vi "FRIC_navX_Internal_I2C_ProcessingLoop.vi"(7 "Device Number":T2, 10 "I2C Bus":T1=enum."I2C MXP", 11 "Rate (4Hz-200Hz)":u8=50 min=4 max=200) -> ()   [LabVIEW 2018]
doc: "This navX VI handles the reading/writing for the navX. All of the good stuff is in here.\nTHIS VI SHOULD NOT BE CALLED BY THE USER!"
uses:
  <vilib>/Rock Robotics/SystemInterfaces/i2clib/i2c_bus.ctl
  _TypeDefs/FRIC_navX_DeviceNumbersTypeDef.ctl
  _TypeDefs/FRIC_navX_ProcessingLoopStatesTypeDef_I2C.ctl
  _TypeDefs/FRIC_navX_I2C Process Loop TypeDef.ctl
  _TypeDefs/Z900_navX_DeviceTypeDef.ctl
  _TypeDefs/Z900_navX_ProtocolTypeDef.ctl
  _TypeDefs/Z900_navX_NotifyPacketTypeDef.ctl
  _TypeDefs/Z900_navX_ActionTypeDef.ctl
  _TypeDefs/Z900_navX_SerialStreamTypeDef.ctl
  _TypeDefs/Z900_navX_IntegrationControlRegisters.ctl
  <vilib>/Rock Robotics/WPI/SPI/WPI_SPIDevRef.ctl
  <vilib>/Rock Robotics/SystemInterfaces/spilib/spi_bus.ctl
  <vilib>/Rock Robotics/WPI/SerialPort/WPI_SerialPort.ctl
  <vilib>/Rock Robotics/WPI/SerialPort/WPI_SerialPortRef.ctl
  <vilib>/Platform/TimedLoop/XDataNode/timing_clust.ctl
  <vilib>/Platform/TimedLoop/XDataNode/nitl_modes.ctl
  <vilib>/Platform/TimedLoop/XDataNode/wakeup.ctl
  _TypeDefs/Z900_navX_DeviceRegisters.ctl
  _TypeDefs/Flags/Z900_navX_Flags_CapabilityTypeDef.ctl
  _Util/Z900_navX_Util_LittleEndian_to_BigEndian.vi
  <vilib>/Rock Robotics/SystemInterfaces/Utilities/FPGA_UtilitiesRead LocalTime.vi
  <vilib>/Platform/TimedLoop/XDataNode/XDataNode.xnode
  <vilib>/Platform/TimedLoop/XDataNode/XDNodeRunTimeDep.lvlib
panel:
  in  "Tab Control":enum32{"Page 1", "Page 2"}(tab)
  in  "Halt":bool
  out "Connected":bool
  out "error":errorcluster
  out "Loop Time":i64
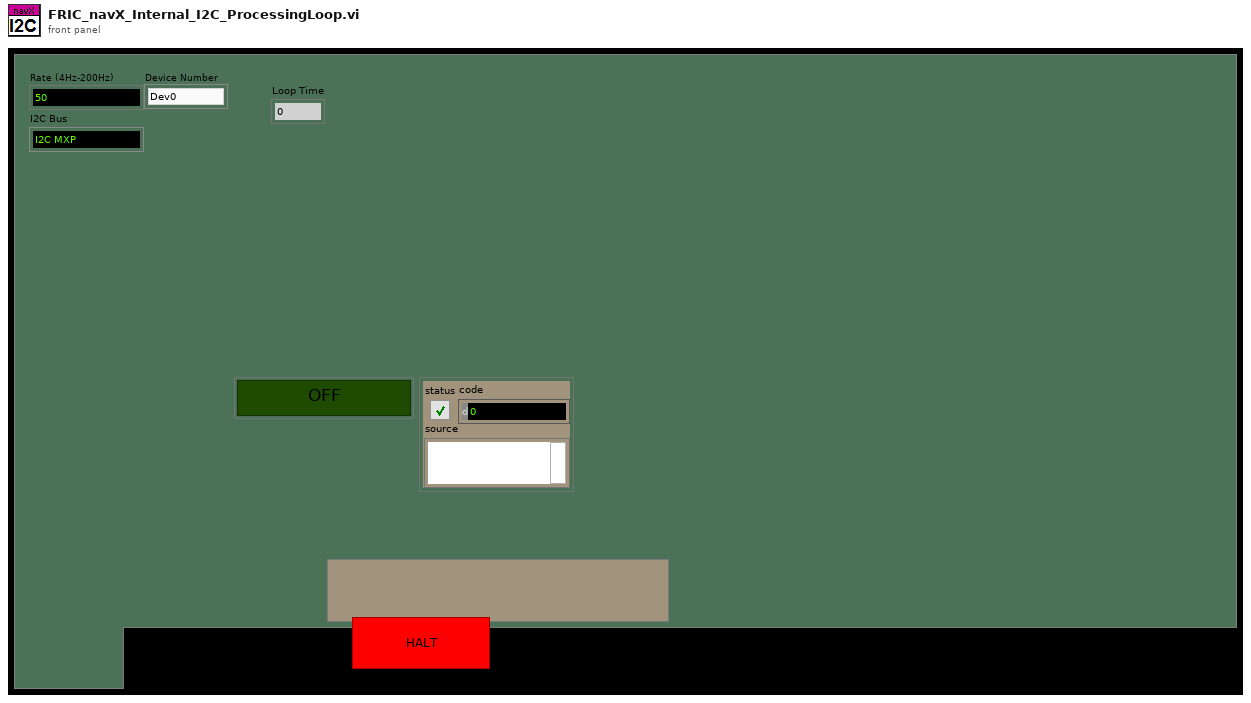
[diagram p1: front panel]
types:
  T1 = typedef "i2c_bus.ctl" = enum16{"I2C On-Board", "I2C MXP", "Invalid"}
  T2 = typedef "FRIC_navX_DeviceNumbersTypeDef.ctl" = enum16{"Dev0", "Dev1", "Dev2", "Dev3"}
  T3 = typedef "FRIC_navX_I2C Process Loop TypeDef.ctl" = cluster{"State Array":T4[], "error":errorcluster, "FPGA Cluster":cluster{"Last Valid FPGA Time":dbl, "Error Count":i32, "Initialized":bool}, "Device Info":T5, "I2CDevRef":cluster{"DevStatus":errorcluster, "Device Address":u8, "Handle":i32, "I2C Bus":T1}, "Registry":u8[], "Command Array":T7[], "Connected?":bool, "navX Device Memory Size":i32, "notification":T8, "Memory Size Set":bool, "SPIDevRef":T11, "navX Serial Open":cluster{"Stream Type":T10, "Serial Port":T13}, "SerialPortRef":T14, "Serial Read Buffer":string, "Serial Write Buffer":string[], "Device Number":T2, "navX SPI Open":cluster{"SPI Bus":T12, "Clock Rate (Hz)":dbl}, "Loop dt":i64, "current time":timestamp, "Loop Time":i64}
  T4 = typedef "FRIC_navX_ProcessingLoopStatesTypeDef_I2C.ctl" = enum16{"Process", "INI", "Check Packets Valid", "Close", "Clear VISA", "Generate Command", "Last Packet Valid", "Open", "Read", "Reset Serial", "Set Termination Char", "Update AE", "Wait", "Write", "Exit"}
  T5 = typedef "Z900_navX_DeviceTypeDef.ctl" = cluster{"Interface":cluster{"Protocol":T6, "Update Rate (4Hz-200Hz)":u8, "navX Open TypeDef":variant}, "Notify Packet":refnum<notifier>, "Loop VI Refnum":refnum<vi>, "Ready to Close Occurrence Refnum":refnum<k4>, "Name":string}
  T6 = typedef "Z900_navX_ProtocolTypeDef.ctl" = enum16{"SERIAL", "I2C", "SPI"}
  T7 = typedef "Z900_navX_IntegrationControlRegisters.ctl" = u8
  T8 = typedef "Z900_navX_NotifyPacketTypeDef.ctl" = cluster{"navX Action":T9, "Data":variant, "Stream Type":T10, "Device Number":T2}
  T9 = typedef "Z900_navX_ActionTypeDef.ctl" = enum16{"None", "Halt", "Normal Read", "Update Serial Protocol", "Update Rate Htz", "Zero-Yaw", "Zero-Displacement", "Zero-Velocity"}
  T10 = typedef "Z900_navX_SerialStreamTypeDef.ctl" = enum16{"YRPH", "Quaterinons", "Gyro/Raw", "AHRS", "AHRSAndPositioning", "AHRSAndPOSTime"}
  T11 = typedef "WPI_SPIDevRef.ctl" = cluster{"DevStatus":errorcluster, "Handle":i32, "SPI Bus":T12}
  T12 = typedef "spi_bus.ctl" = enum16{"SPI On-Board, CS0", "SPI On-Board, CS1", "SPI On-Board, CS2", "SPI On-Board, CS3", "SPI MXP", "Invalid"}
  T13 = typedef "WPI_SerialPort.ctl" = enum16{"Onboard RS-232", "MXP TTL", "USB 1", "USB 2"}
  T14 = typedef "WPI_SerialPortRef.ctl" = cluster{"DevStatus":errorcluster, "Serial Port Name":refnum<visa-resource-name>}
  T15 = typedef "XDNodeRunTimeDep.lvlib/timing_clust.ctl" = cluster{"Expected End [f-1]":u64, "Actual End [f-1]":u64, "Finished Late? [f-1]":bool, "Expected End [i-1]":u64, "Actual End [i-1]":u64, "Finished Late? [i-1]":bool, "Expected Start [i]":u64, "Actual Start [i]":u64, "Expected Start [f]":u64, "Actual Start [f]":u64, "Source Name":string, "Structure Name":string, "Period":i64, "Deadline":i64, "Offset":i64, "Start":i64, "Priority":i32, "Timeout":i32, "Mode":T16, "Wakeup Reason":T17, "Error":errorcluster, "Source Type":string, "Secondary Source Type":string, "Global End Time":u64, "Global Start Time":u64, "Frame Duration":u64, "Iteration Duration":u64, "Assigned CPU":i32, "I/O Scan Engine Mode":u32}
  T16 = typedef "XDNodeRunTimeDep.lvlib/nitl_modes.ctl" = enum32{"No Change", "Process missed periods, maintain original phase", "Discard missed periods, maintain original phase", "Process missed periods, ignore original phase", "Discard missed periods, ignore original phase"}
  T17 = typedef "XDNodeRunTimeDep.lvlib/wakeup.ctl" = enum32{"Normal", "Aborted", "Asynchronous wakeup", "Timing source error", "Timed loop error", "Timeout"}
  T18 = typedef "Z900_navX_DeviceRegisters.ctl" = u8
  T19 = typedef "Z900_navX_Flags_CapabilityTypeDef.ctl" = u16
  T20 = cluster{"DevStatus":errorcluster, "Device Address":u8, "Handle":i32, "I2C Bus":T1}
  T21 = cluster{"Last Valid FPGA Time":dbl, "Error Count":i32, "Initialized":bool}
  T22 = typedef "WPI_I2CDevRef.ctl" = cluster{"DevStatus":errorcluster, "Device Address":u8, "Handle":i32, "I2C Bus":T1}
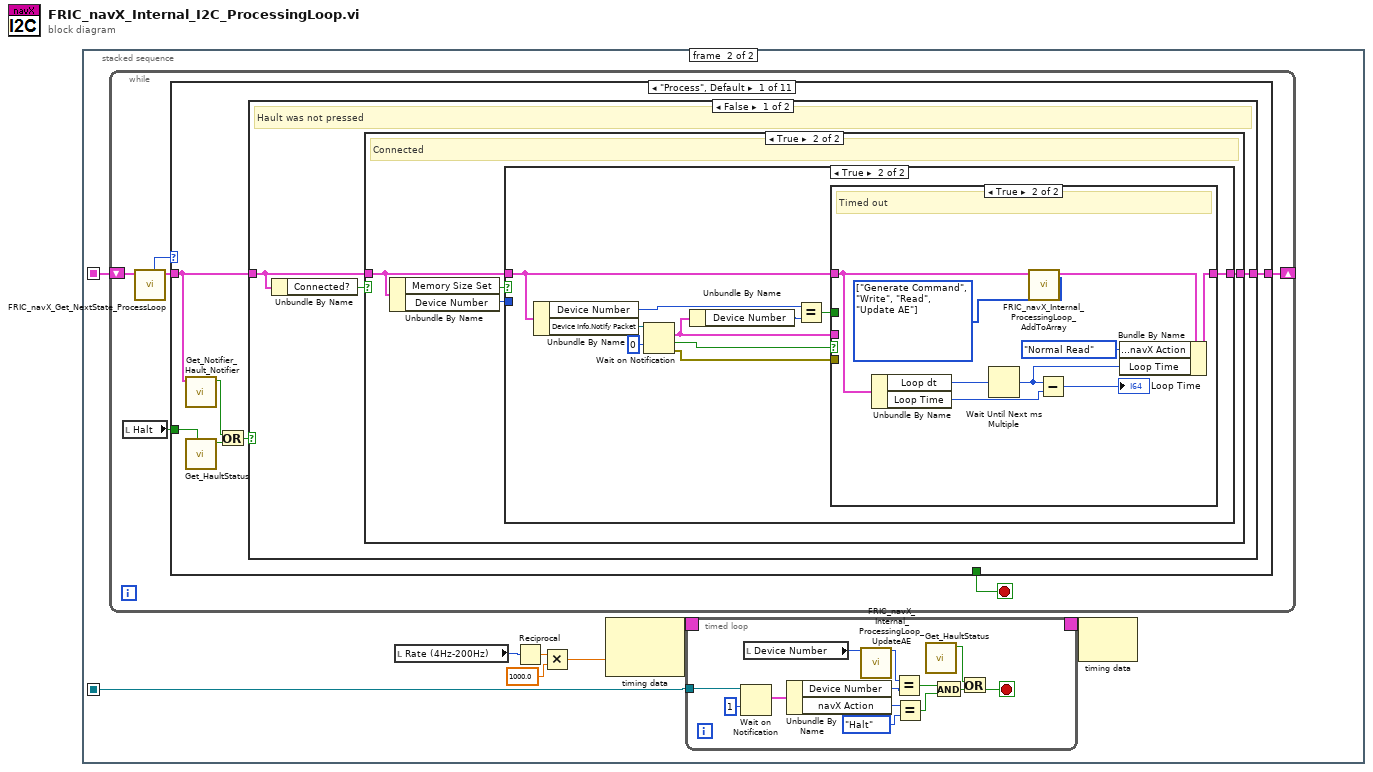
[diagram p0: block diagram]
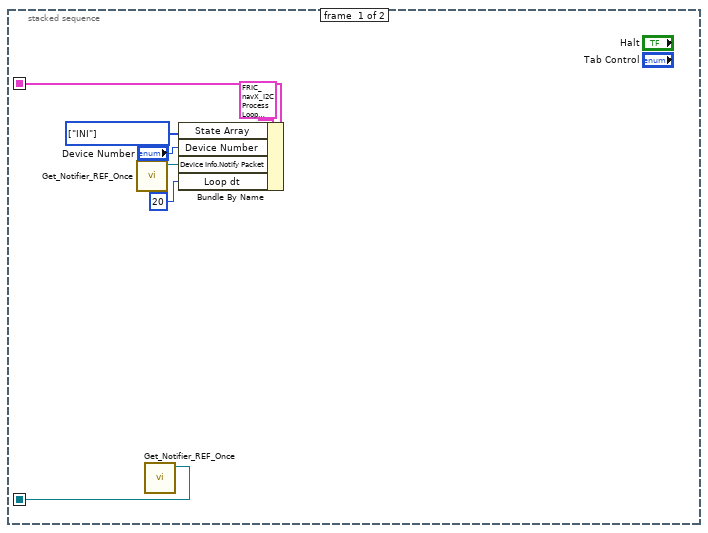
[diagram p2: hidden frame]
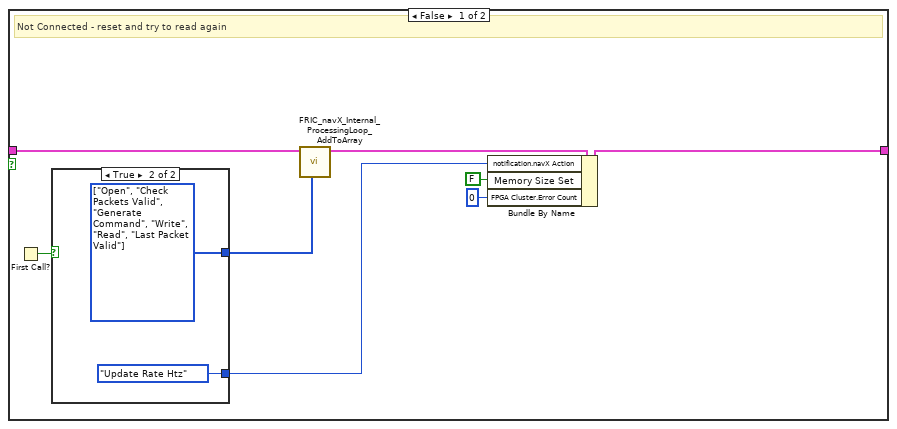
[diagram p3: hidden frame]
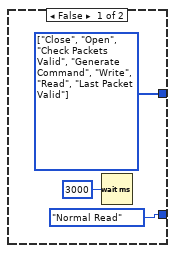
[diagram p4: hidden frame]
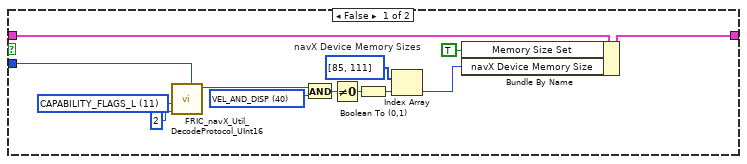
[diagram p5: hidden frame]
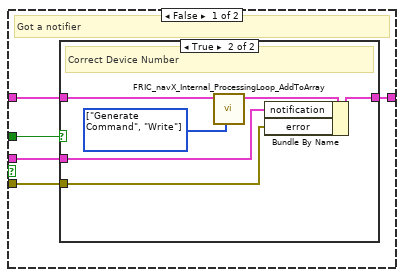
[diagram p6: hidden frame]
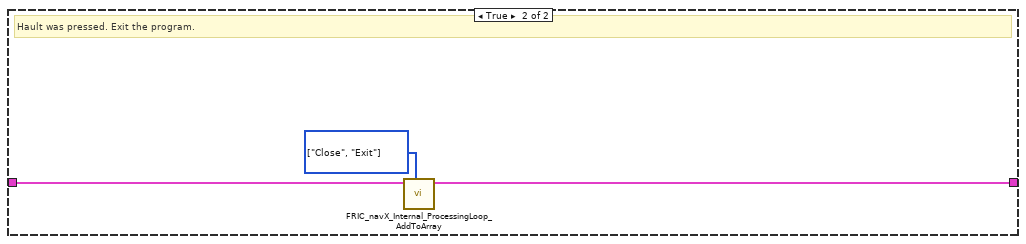
[diagram p8: hidden frame]
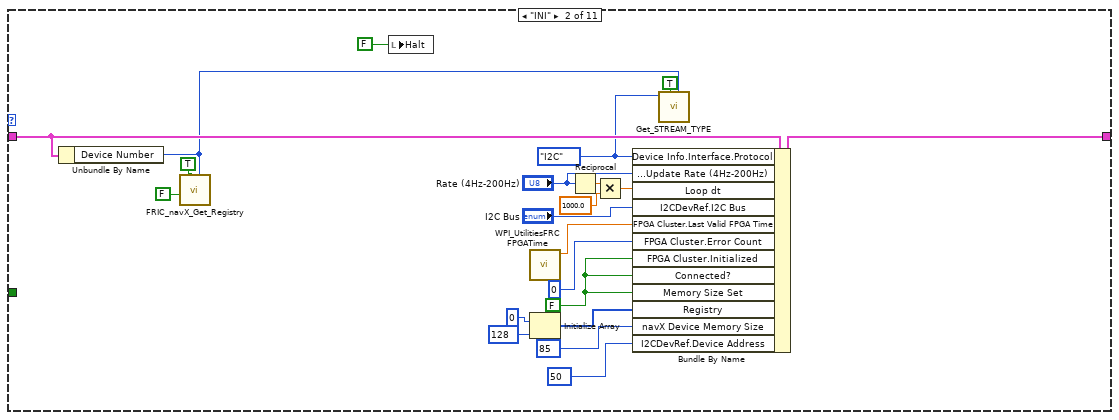
[diagram p9: hidden frame]
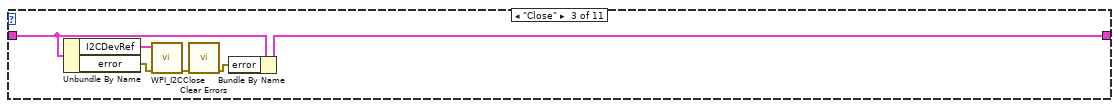
[diagram p10: hidden frame]
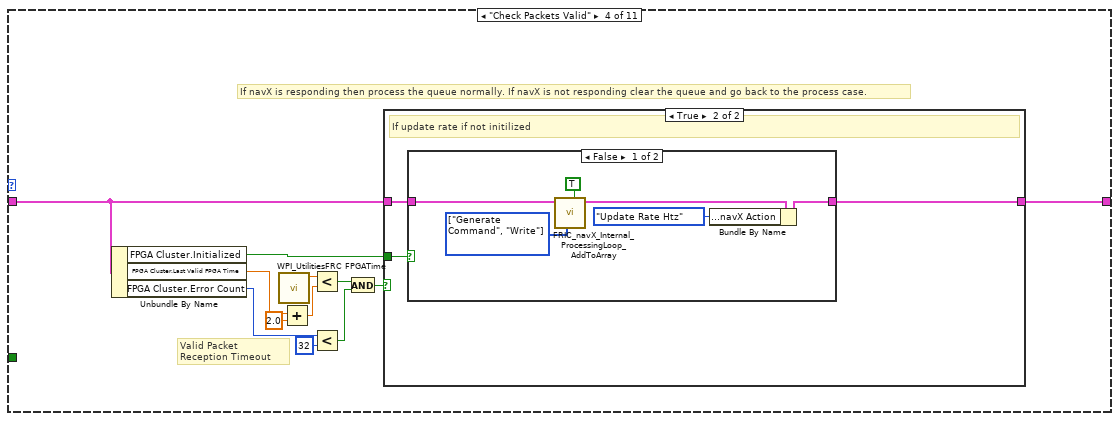
[diagram p11: hidden frame]
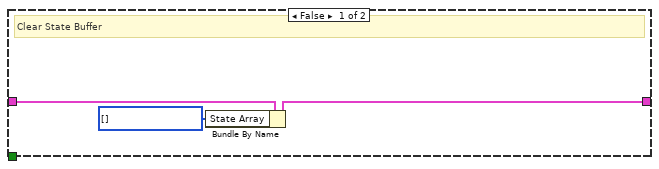
[diagram p12: hidden frame]
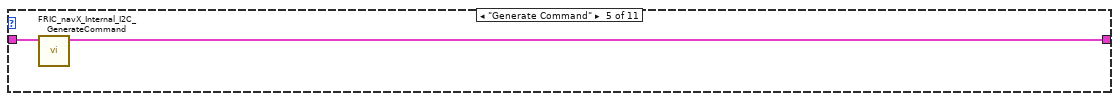
[diagram p14: hidden frame]
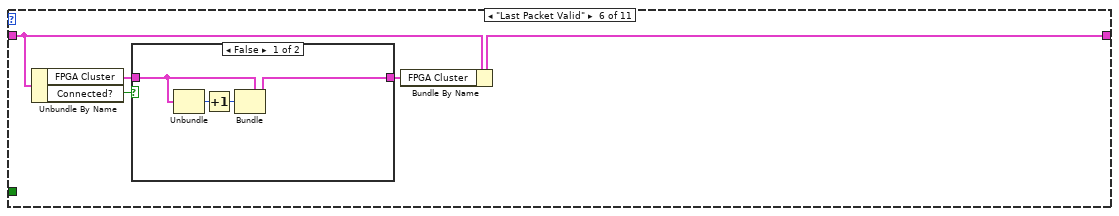
[diagram p15: hidden frame]
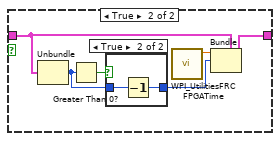
[diagram p16: hidden frame]
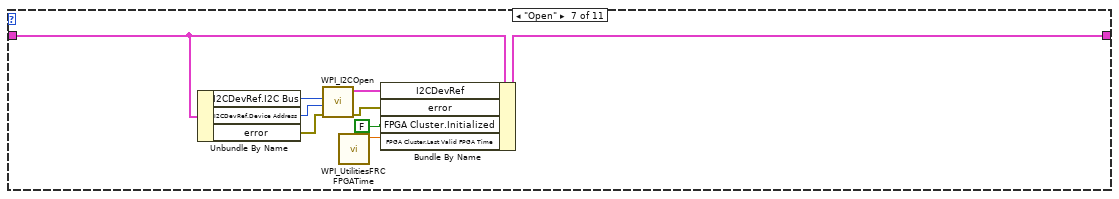
[diagram p18: hidden frame]
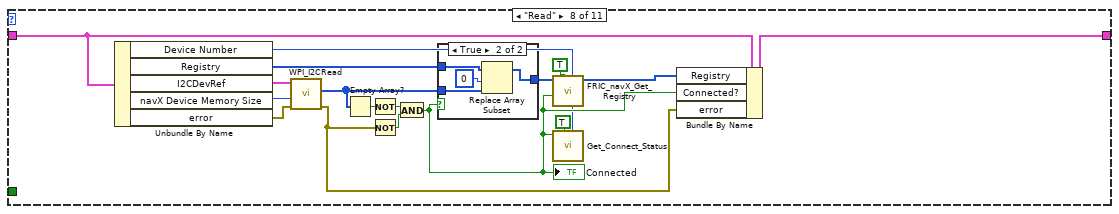
[diagram p19: hidden frame]
diagram:
  n1 = stacked-sequence {
    seq-local: [w7 _] -> [_ w15]
    seq-local: [w1 _] -> [_ w8]
    frame #0 {
      w5 = T4[] [enum."INI"] items=["Process", "INI", "Check Packets Valid", "Close", "Clear VISA", "Generate Command", "Last Packet Valid", "Open", "Read", "Reset Serial", "Set Termination Char", "Update AE", "Wait", "Write", "Exit"] ("State Array")
      n2 = call "Get_Notifier_REF_Once.vi"() -> ("notifier ref out"=w3:refnum<notifier>)  [unwired: 10 in, 1 out]
      n3 = call "Get_Notifier_REF_Once.vi"() -> ("notifier ref out"=w1:refnum<notifier>)  [unwired: 10 in, 1 out]
      n4 = Bundle By Name(cluster=T3 {"State Array"=[enum."INI", enum."Open"], "error"={"status"=FALSE, "code"=0, "source"=""}, "FPGA Cluster"={"Last Valid FPGA Time"=0.0, "Error Count"=0, "Initialized"=FALSE}, "Device Info"={"Interface"={"Protocol"=enum."SERIAL", "Update Rate (4Hz-200Hz)"=4, "navX Open TypeDef"=variant}, "Notify Packet"=refnum, "Loop VI Refnum"=refnum, "Ready to Close Occurrence Refnum"=refnum, "Name"=""}, "I2CDevRef"={"DevStatus"={"status"=FALSE, "code"=0, "source"=""}, "Device Address"=0, "Handle"=0, "I2C Bus"=enum."Invalid"}, "Registry"=[], "Command Array"=[214, 32], "Connected?"=FALSE, "navX Device Memory Size"=85, "notification"={"navX Action"=enum."None", "Data"=variant, "Stream Type"=enum."YRPH", "Device Number"=enum."Dev0"}, "Memory Size Set"=FALSE, "SPIDevRef"={"DevStatus"={"status"=FALSE, "code"=0, "source"=""}, "Handle"=0, "SPI Bus"=enum."SPI On-Board, CS0"}, "navX Serial Open"={"Stream Type"=enum."YRPH", "Serial Port"=enum."Onboard RS-232"}, "SerialPortRef"={"DevStatus"={"status"=FALSE, "code"=0, "source"=""}, "Serial Port Name"=""}, "Serial Read Buffer"="", "Serial Write Buffer"=[], "Device Number"=enum."Dev0", "navX SPI Open"={"SPI Bus"=enum."SPI MXP", "Clock Rate (Hz)"=500000.0}, "Loop dt"=0, "current time"=timestamp(0 s since 1904-01-01), "Loop Time"=0} ("I2C Process Loop TypeDef"), "State Array"=w5, "Device Number"="Device Number", "Device Info.Notify Packet"=w3, "Loop dt"=i64 20) -> (w7:T3)
    }
    frame #1 {
      n5 = while {
        shift-right: [w35] -> _
        shift-left: w15 -> [w38]
        stop <- w39 stop-if-true
        n6 = local read "Halt"() -> (w34:bool)
        n7 = call "FRIC_navX_Get_NextState_ProcessLoop.vi"("I2C Process Loop TypeDef (in)"=w38) -> ("I2C Process Loop TypeDef (out)"=w37:T3, "Current State"=w36:T4)  [unwired: 9 in]
        n8 = case shown="\"Process\", Default" w36 {
          tunnel: [_ _ _ _ _ _ _ _ _ w223 _] -> w39
          tunnel: w37 -> [w44 w123 w137 w144 w166 w170 w192 w205 w221 w225 w233]
          tunnel: [w45 w129 w136 w145 w165 w169 w191 w204 w222 w225 w233] -> w35
          tunnel: w34 -> [w42 _ _ _ _ _ _ _ _ _ _]
          frame "Process", Default {
            n9 = call "Get_Notifier_Hault_Notifier.vi"("Process Loop TypeDef (in)"=w44) -> ("Hault Notifier"=w41:bool)  [unwired: 10 in]
            n10 = call "Get_HaultStatus.vi"("Update"=w42) -> ("Hault"=w40:bool)  [unwired: 10 in]
            n11 = Or(x=w41, y=w40) -> (x .or. y?=w43:bool)
            n12 = case shown="False" w43 {
              tunnel: [w48 w111] -> w45
              tunnel: w44 -> [w46 w112]
              frame False {
                # "Hault was not pressed"
                n13 = Unbundle By Name(w46) -> ("Connected?"=w47:bool)
                n14 = case shown="True" w47 {
                  tunnel: w46 -> [w56 w64]
                  tunnel: [w53 w65] -> w48
                  frame False {
                    # "Not Connected - reset and try to read again"
                    n15 = First Call?() -> (First Call?: T/F=w50:bool)
                    n16 = case shown="True" w50 {
                      tunnel: [w59 w61] -> w55
                      tunnel: [Z900_navX_ActionTypeDef."Normal Read" ("notification.navX Action") Z900_navX_ActionTypeDef."Update Rate Htz" ("notification.navX Action")] -> w49
                      frame False {
                        w59 = T4[] [enum."Close", enum."Open", enum."Check Packets Valid", enum."Generate Command", enum."Write", enum."Read", enum."Last Packet Valid"] items=["Process", "INI", "Check Packets Valid", "Close", "Clear VISA", "Generate Command", "Last Packet Valid", "Open", "Read", "Reset Serial", "Set Termination Char", "Update AE", "Wait", "Write", "Exit"]
                        n17 = Wait (ms)(milliseconds to wait=u32 3000) -> ()  [unwired: 1 out]
                      }
                      frame True {
                        w61 = T4[] [enum."Open", enum."Check Packets Valid", enum."Generate Command", enum."Write", enum."Read", enum."Last Packet Valid"] items=["Process", "INI", "Check Packets Valid", "Close", "Clear VISA", "Generate Command", "Last Packet Valid", "Open", "Read", "Reset Serial", "Set Termination Char", "Update AE", "Wait", "Write", "Exit"]
                      }
                    }
                    n18 = call "FRIC_navX_Internal_ProcessingLoop_AddToArray.vi"("States Array"=w55, "I2C Process Loop TypeDef (in)"=w56) -> ("I2C Process Loop TypeDef (out)"=w54:T3)  [unwired: 9 in]
                    n19 = Bundle By Name(cluster=w54, "notification.navX Action"=w49, "Memory Size Set"=FALSE, "FPGA Cluster.Error Count"=0) -> (w53:T3)
                  }
                  frame True {
                    # "Connected"
                    n20 = Unbundle By Name(w64) -> ("Memory Size Set"=w63:bool, "Device Number"=w62:T2)
                    n21 = case shown="True" w63 {
                      tunnel: [w77 w86] -> w65
                      tunnel: w64 -> [w78 w84]
                      tunnel: w62 -> [w66 _]
                      frame False {
                        w76 = T18 11 items=["WHOAMI"=0, "HW_REV"=1, "FW_VER_MAJOR"=2, "FW_VER_MINOR"=3, "UPDATE_RATE_HZ"=4, "ACCEL_FSR_G"=5, "GYRO_FSR_DPS"=6, "OP_STATUS"=8, "CAL_STATUS"=9, "SELFTEST_STATUS"=10, "CAPABILITY_FLAGS_L"=11, "CAPABILITY_FLAGS_H"=12, "SENSOR_STATUS"=16, "TIMESTAMP"=18, "YAW"=22, "ROLL"=24, "PITCH"=26, "HEADING"=28, "FUSED_HEADING"=30, "ALTITUDE_I"=32, "ALTITUDE_D"=34, "LINERA_ACC_X"=36, "LINERA_ACC_Y"=38, "LINERA_ACC_Z"=40, "QUAT_W"=42, "QUAT_X"=44, "QUAT_Y"=46, "QUAT_Z"=48, "MPU_TEMP_C"=50, "GYRO_X"=52, "GYRO_Y"=54, "GYRO_Z"=56, "ACC_X"=58, "ACC_Y"=60, "ACC_Z"=62, "MAG_X"=64, "MAG_Y"=66, "MAG_Z"=68, "PRESSURE_I"=70, "PRESSURE_D"=72, "PRESSURE_TEMP"=74, "YAW_OFFSET"=76, "QUAT_OFFSET_W"=78, "QUAT_OFFSET_X"=80, "QUAT_OFFSET_Y"=82, "QUAT_OFFSET_Z"=84, "INTEGRATION_CONTROL"=86, "VELOCITY_X"=88, "VELOCITY_Y"=92, "VELOCITY_Z"=96, "DISPLACMENT_X"=100, "DISPLACMENT_Y"=104, "DISPLACEMENT_Z"=108] ("Device Register")
                        w71 = T19 40 items=["OMNIMOUNT"=4, "OMNIMOUNT_CONFIG_MASK"=38, "VEL_AND_DISP"=40, "YAW_RESET"=80] ("Capability Flag")
                        w72 = i32[] [85, 111]  # navX Device Memory Sizes
                        n22 = call "FRIC_navX_Util_DecodeProtocol_UInt16.vi"("Device Number"=w66, "length"=2, "Device Register"=w76) -> ("Value"=w69:u16)  [unwired: 8 in]
                        n23 = And(x=w69, y=w71) -> (x .and. y?=w70:T19)
                        n24 = Not Equal To 0?(x=w70) -> (x != 0?=w73:bool)
                        n25 = Boolean To (0,1)(Boolean=w73) -> (0, 1=w74:i16)
                        n26 = Index Array(array=w72, index=w74) -> (element=w68:i32)
                        n27 = Bundle By Name(cluster=w78, "Memory Size Set"=TRUE, "navX Device Memory Size"=w68) -> (w77:T3)
                      }
                      frame True {
                        n28 = Unbundle By Name(w84) -> ("Device Number"=w81:T2, "Device Info.Notify Packet"=w88:refnum<notifier>)
                        n29 = Wait on Notification(notifier=w88, timeout in ms (-1)=0) -> (notification=w82:T8, timed out?=w83:bool, error out=w85:errorcluster)  [unwired: 2 in, 1 out]
                        n30 = Unbundle By Name(w82) -> ("Device Number"=w80:T2)
                        n31 = Equal?(x=w81, y=w80) -> (x = y?=w79:bool)
                        n32 = case shown="True" w83 {
                          tunnel: w84 -> [w93 w106]
                          tunnel: [w92 w108] -> w86
                          tunnel: w82 -> [w91 _]
                          tunnel: w85 -> [w90 _]
                          tunnel: w79 -> [w89 _]
                          frame False {
                            # "Got a notifier"
                            n33 = case shown="True" w89 {
                              tunnel: w93 -> [w94 w100]
                              tunnel: [w94 w99] -> w92
                              tunnel: w91 -> [_ w98]
                              tunnel: w90 -> [_ w95]
                              frame False {
                              }
                              frame True {
                                w96 = T4[] [enum."Generate Command", enum."Write"] items=["Process", "INI", "Check Packets Valid", "Close", "Clear VISA", "Generate Command", "Last Packet Valid", "Open", "Read", "Reset Serial", "Set Termination Char", "Update AE", "Wait", "Write", "Exit"] ("States Array")
                                # "Correct Device Number"
                                n34 = call "FRIC_navX_Internal_ProcessingLoop_AddToArray.vi"("States Array"=w96, "I2C Process Loop TypeDef (in)"=w100) -> ("I2C Process Loop TypeDef (out)"=w97:T3)  [unwired: 9 in]
                                n35 = Bundle By Name(cluster=w97, "notification"=w98, "error"=w95) -> (w99:T3)
                              }
                            }
                          }
                          frame True {
                            w105 = T4[] [enum."Generate Command", enum."Write", enum."Read", enum."Update AE"] items=["Process", "INI", "Check Packets Valid", "Close", "Clear VISA", "Generate Command", "Last Packet Valid", "Open", "Read", "Reset Serial", "Set Termination Char", "Update AE", "Wait", "Write", "Exit"]
                            # "Timed out"
                            n36 = Unbundle By Name(w106) -> ("Loop dt"=w104:i64, "Loop Time"=w102:i64)
                            n37 = Wait Until Next ms Multiple(millisecond multiple=w104) -> (millisecond timer value=w103:u32)
                            n38 = call "FRIC_navX_Internal_ProcessingLoop_AddToArray.vi"("States Array"=w105, "I2C Process Loop TypeDef (in)"=w106) -> ("I2C Process Loop TypeDef (out)"=w109:T3)  [unwired: 9 in]
                            n39 = Subtract(x=w103, y=w102) -> (x-y=→"Loop Time":i64)
                            n40 = Bundle By Name(cluster=w109, "notification.navX Action"=Z900_navX_ActionTypeDef."Normal Read", "Loop Time"=w103) -> (w108:T3)
                          }
                        }
                      }
                    }
                  }
                }
              }
              frame True {
                w110 = T4[] [enum."Close", enum."Exit"] items=["Process", "INI", "Check Packets Valid", "Close", "Clear VISA", "Generate Command", "Last Packet Valid", "Open", "Read", "Reset Serial", "Set Termination Char", "Update AE", "Wait", "Write", "Exit"] ("States Array")
                # "Hault was pressed. Exit the program."
                n41 = call "FRIC_navX_Internal_ProcessingLoop_AddToArray.vi"("States Array"=w110, "I2C Process Loop TypeDef (in)"=w112) -> ("I2C Process Loop TypeDef (out)"=w111:T3)  [unwired: 9 in]
              }
            }
          }
          frame "INI" {
            w113 = Z900_navX_ProtocolTypeDef."I2C" ("Protocol")
            w127 = FALSE ("Initialized")
            n42 = Unbundle By Name(w123) -> ("Device Number"=w114:T2)
            n43 = call "FRIC_navX_Get_Registry.vi"("Device Number"=w114, "Update"=TRUE, "Connected?"=FALSE) -> ()  [unwired: 7 in, 2 out]
            n44 = local write "Halt"(FALSE ("Halt")) -> ()
            n45 = call <vilib>:"WPI_UtilitiesFRC FPGATime.vi"() -> ("FPGA Time"=w131:dbl)  [unwired: 10 in, 1 out]
            n46 = Initialize Array(u8 0 ("Received Data"), 128 ("hex")) -> (w126:u8[])
            n47 = Reciprocal(x="Rate (4Hz-200Hz)") -> (1/x=w119:dbl)
            n48 = Multiply(x=w119, y=1000.0) -> (x*y=w118:dbl)
            n49 = Bundle By Name(cluster=w123, "Device Info.Interface.Protocol"=w113, "Device Info.Interface.Update Rate (4Hz-200Hz)"="Rate (4Hz-200Hz)", "Loop dt"=w118, "I2CDevRef.I2C Bus"="I2C Bus", "FPGA Cluster.Last Valid FPGA Time"=w131, "FPGA Cluster.Error Count"=0 ("Error Count"), "FPGA Cluster.Initialized"=w127, "Connected?"=w127, "Memory Size Set"=w127, "Registry"=w126, "navX Device Memory Size"=85 ("hex"), "I2CDevRef.Device Address"=50 ("hex")) -> (w129:T3)
            n50 = call "Get_STREAM_TYPE.vi"("Device Number"=w114, "Update"=TRUE, "Protocol (in)"=w113) -> ()  [unwired: 8 in, 1 out]
          }
          frame "Close" {
            n51 = Unbundle By Name(w137) -> ("I2CDevRef"=w139:T20, "error"=w138:errorcluster)
            n52 = call <vilib>:"WPI_I2CClose.vi"("error in (no error)"=w138, "I2CDevRef"=w139) -> ("error out"=w135:errorcluster)  [unwired: 9 in]
            n53 = call <vilib>:"Clear Errors.vi"("error in (no error)"=w135) -> ("error out"=w134:errorcluster)  [unwired: 5 in, 1 out]
            n54 = Bundle By Name(cluster=w137, "error"=w134) -> (w136:T3)
          }
          frame "Check Packets Valid" {
            # "If navX is responding then process the queue normally. If navX is not responding clear the queue and go back to the process case."
            # "Valid Packet Reception Timeout"
            n55 = Unbundle By Name(w144) -> ("FPGA Cluster.Initialized"=w142:bool, "FPGA Cluster.Last Valid FPGA Time"=w143:dbl, "FPGA Cluster.Error Count"=w141:i32)
            n56 = call <vilib>:"WPI_UtilitiesFRC FPGATime.vi"() -> ("FPGA Time"=w149:dbl)  [unwired: 10 in, 1 out]
            n57 = Add(x=w143, y=2.0) -> (x+y=w150:dbl)
            n58 = Less?(x=w149, y=w150) -> (x < y?=w147:bool)
            n59 = Less?(x=w141, y=32) -> (x < y?=w146:bool)
            n60 = And(x=w147, y=w146) -> (x .and. y?=w140:bool)
            n61 = case shown="True" w140 {
              tunnel: w144 -> [w154 w157]
              tunnel: [w153 w156] -> w145
              tunnel: w142 -> [_ w155]
              frame False {
                w152 = T4[] [] items=["Process", "INI", "Check Packets Valid", "Close", "Clear VISA", "Generate Command", "Last Packet Valid", "Open", "Read", "Reset Serial", "Set Termination Char", "Update AE", "Wait", "Write", "Exit"] ("f")
                # "Clear State Buffer"
                n62 = Bundle By Name(cluster=w154, "State Array"=w152) -> (w153:T3)
              }
              frame True {
                # "If update rate if not initilized"
                n63 = case shown="False" w155 {
                  tunnel: w157 -> [w162 w164]
                  tunnel: [w160 w164] -> w156
                  frame False {
                    w158 = T4[] [enum."Generate Command", enum."Write"] items=["Process", "INI", "Check Packets Valid", "Close", "Clear VISA", "Generate Command", "Last Packet Valid", "Open", "Read", "Reset Serial", "Set Termination Char", "Update AE", "Wait", "Write", "Exit"] ("f")
                    n64 = call "FRIC_navX_Internal_ProcessingLoop_AddToArray.vi"("Add to beginning"=TRUE, "States Array"=w158, "I2C Process Loop TypeDef (in)"=w162) -> ("I2C Process Loop TypeDef (out)"=w161:T3)  [unwired: 8 in]
                    n65 = Bundle By Name(cluster=w161, "notification.navX Action"=Z900_navX_ActionTypeDef."Update Rate Htz") -> (w160:T3)
                  }
                  frame True {
                  }
                }
              }
            }
          }
          frame "Generate Command" {
            n66 = call "FRIC_navX_Internal_I2C_GenerateCommand.vi"("I2C Process Loop TypeDef (in)"=w166) -> ("I2C Process Loop TypeDef (out)"=w165:T3)  [unwired: 10 in]
          }
          frame "Last Packet Valid" {
            n67 = Unbundle By Name(w170) -> ("FPGA Cluster"=w171:T21, "Connected?"=w167:bool)
            n68 = case shown="False" w167 {
              tunnel: [w174 w181] -> w168
              tunnel: w171 -> [w173 w177]
              frame False {
                n69 = Unbundle(w173) -> ("Error Count"=w172:i32)  [unwired: 2 out]
                n70 = Increment(x=w172) -> (x+1=w175:i32)
                n71 = Bundle(cluster=w173, "Error Count"=w175) -> (w174:T21)  [unwired: 2 in]
              }
              frame True {
                n72 = Unbundle(w177) -> ("Error Count"=w176:i32)  [unwired: 2 out]
                n73 = Greater Than 0?(x=w176) -> (x > 0?=w179:bool)
                n74 = case shown="True" w179 {
                  tunnel: [w182 w184] -> w178
                  tunnel: w176 -> [w182 w183]
                  frame False {
                  }
                  frame True {
                    n75 = Decrement(x=w183) -> (x-1=w184:i32)
                  }
                }
                n76 = call <vilib>:"WPI_UtilitiesFRC FPGATime.vi"() -> ("FPGA Time"=w180:dbl)  [unwired: 10 in, 1 out]
                n77 = Bundle(cluster=w177, "Last Valid FPGA Time"=w180, "Error Count"=w178) -> (w181:T21)  [unwired: 1 in]
              }
            }
            n78 = Bundle By Name(cluster=w170, "FPGA Cluster"=w168) -> (w169:T3)
          }
          frame "Open" {
            n79 = Unbundle By Name(w192) -> ("I2CDevRef.I2C Bus"=w186:T1, "I2CDevRef.Device Address"=w185:u8, "error"=w187:errorcluster)
            n80 = call <vilib>:"WPI_I2COpen.vi"("error in"=w187, "Device Address"=w185, "I2C Bus"=w186) -> ("error out"=w190:errorcluster, "I2CDevRef"=w193:T22)  [unwired: 7 in]
            n81 = call <vilib>:"WPI_UtilitiesFRC FPGATime.vi"() -> ("FPGA Time"=w188:dbl)  [unwired: 10 in, 1 out]
            n82 = Bundle By Name(cluster=w192, "I2CDevRef"=w193, "error"=w190, "FPGA Cluster.Initialized"=FALSE ("Initialized"), "FPGA Cluster.Last Valid FPGA Time"=w188) -> (w191:T3)
          }
          frame "Read" {
            n83 = Unbundle By Name(w205) -> ("Device Number"=w197:T2, "Registry"=w194:u8[], "I2CDevRef"=w208:T20, "navX Device Memory Size"=w206:i32, "error"=w207:errorcluster)
            n84 = call <vilib>:"WPI_I2CRead.vi"("error in (no error)"=w207, "I2CBytesToRead"=w206, "I2CDevRef"=w208) -> ("error out"=w195:errorcluster, "Data Out"=w202:u8[])  [unwired: 6 in, 1 out]
            n85 = Empty Array?(array=w202) -> (empty?=w201:bool)
            n86 = Not(x=w201) -> (.not. x?=w200:bool)
            n87 = Not(x=w195) -> (.not. x?=w196:bool)
            n88 = And(x=w200, y=w196) -> (x .and. y?=w198:bool)
            "Connected" <- w198
            n89 = case shown="True" w198 {
              tunnel: w194 -> [w211 w215]
              tunnel: [w211 w214] -> w210
              tunnel: w202 -> [_ w213]
              frame False {
              }
              frame True {
                n90 = Replace Array Subset(array=w215, new element=w213, index=u8 0 ("hex")) -> (w214:u8[])
              }
            }
            n91 = call "FRIC_navX_Get_Registry.vi"("Device Number"=w197, "Update"=TRUE, "Connected?"=w198, "Registry (in)"=w210) -> ("Registry (out)"=w203:u8[])  [unwired: 6 in, 1 out]
            n92 = call "Get_Connect_Status.vi"("Device Number"=w197, "Update"=TRUE, "Connected"=w198) -> ()  [unwired: 8 in, 1 out]
            n93 = Bundle By Name(cluster=w205, "Registry"=w203, "Connected?"=w198, "error"=w195) -> (w204:T3)
          }
          frame "Write" {
            n94 = Unbundle By Name(w221) -> ("I2CDevRef.Handle"=w217:i32, "I2CDevRef.Device Address"=w216:u8, "Command Array"=w220:T7[], "I2CDevRef.DevStatus"=w218:errorcluster)
            n95 = call <vilib>:"i2clib_write.vi"("error in (no error)"=w218, "send_data"=w220, "dev_addr"=w216, "I2C Reference"=w217) -> ("error out"=w219:errorcluster)  [unwired: 6 in, 1 out]
            n96 = Bundle By Name(cluster=w221, "error"=w219) -> (w222:T3)
          }
          frame "Exit" {
            n97 = Unbundle By Name(w225) -> ("Device Info"=w224:T5)
            n98 = in-place {
              in-place-border: w224 -> [w228]
              in-place-border: [TRUE] -> w223
              # "Set Occurence of Close"
              n99 = Unbundle By Name(w228) -> ("Ready to Close Occurrence Refnum"=w229:refnum<k4>)
              n100 = local write "Halt"(FALSE ("Halt")) -> ()
              n101 = Set Occurrence(w229) -> ()
            }
          }
          frame "Update AE" {
            n102 = Unbundle By Name(w233) -> ("Device Number"=w231:T2, "error"=w232:errorcluster)
            "error" <- w232
            n103 = call "Get_Error_Status.vi"("Device Number"=w231, "Update"=TRUE, "error in"=w232) -> ()  [unwired: 8 in, 1 out]
          }
        }
      }
      n104 = local read "Rate (4Hz-200Hz)"() -> (w13:u8)
      n105 = Reciprocal(x=w13) -> (1/x=w14:dbl)
      n106 = Multiply(x=w14, y=1000.0) -> (x*y=w9:dbl)
      n107 = node-c288(w9) -> (w11:T15)  [unwired: 1 in]
      n108 = timed-loop {
        timing: w11 -> [_]
        timing-out: [_] -> w10
        tunnel: w8 -> [w24]
        stop <- w17 stop-if-true
        n109 = Wait on Notification(notifier=w24, timeout in ms (-1)=1) -> (notification=w23:T8)  [unwired: 2 in, 3 out]
        n110 = local read "Device Number"() -> (w21:T2)
        n111 = Unbundle By Name(w23) -> ("Device Number"=w22:T2, "navX Action"=w26:T9)
        n112 = call "FRIC_navX_Internal_ProcessingLoop_UpdateAE.vi"("Device Number"=w21) -> ()  [unwired: 15 in]
        n113 = Equal?(x=w21, y=w22) -> (x = y?=w20:bool)
        n114 = Equal?(x=w26, y=Z900_navX_ActionTypeDef."Halt") -> (x = y?=w19:bool)
        n115 = call "Get_HaultStatus.vi"() -> ("Hault"=w16:bool)  [unwired: 11 in]
        n116 = And(x=w20, y=w19) -> (x .and. y?=w18:bool)
        n117 = Or(x=w16, y=w18) -> (x .or. y?=w17:bool)
      }
      n118 = node-c288(w10) -> ()  [unwired: 1 out]
    }
  }
